vi "Serial Read to CRLF.vi"(8 "error in":errorcluster, 9 "timeout (ms)":i32, 10 "bytes to read":u32, 11 "Visa Resource":refnum<visa-resource-name>) -> (0 "error out":errorcluster, 1 "timed out?":bool, 3 "data":u8[](array[numeric]))   [LabVIEW 2021, in "Serial Shared Components.lvlib"]
doc: "Performs a read on the serial port."
uses:
  Serial Shared Components.lvlib
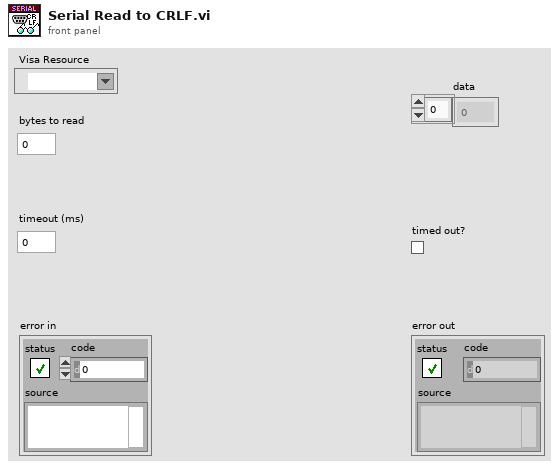
[diagram p1: front panel]
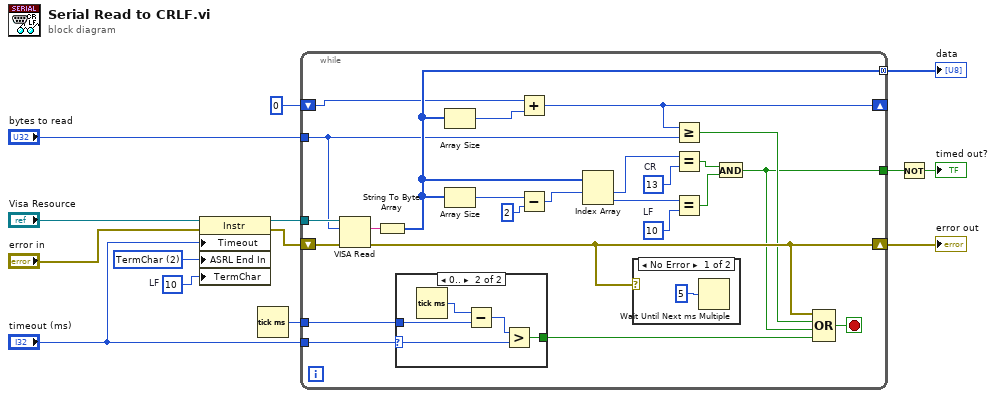
[diagram p0: block diagram]
diagram:
  w10 = u8 10  # LF
  w11 = u16 2 items=["None", "Last Bit", "TermChar"] ("Serial Settings:End Mode for Reads")
  n1 = property class="Instr"(reference="Visa Resource", error in="error in", "Timeout"="timeout (ms)", "ASRL End In"=w11, "TermChar"=w10) -> (reference out=w9:refnum<visa-resource-name>, error out=w8:errorcluster)
  n2 = Tick Count (ms)() -> (millisecond timer value=w13:u32)
  n3 = while {
    tunnel: w13 -> [w36]
    shift-right: [w34] -> w1
    shift-left: w8 -> [w38]
    tunnel: "bytes to read" -> [w22]
    tunnel: w9 -> [w35]
    tunnel: [w16] -> w3
    tunnel: "timeout (ms)" -> [w25]
    tunnel: [w24] -> w2 mode=concatenating
    shift-right: [w23] -> _
    shift-left: 0 -> [w18]
    stop <- w37 stop-if-true
    w28 = u8 10  # LF
    w15 = u8 13  # CR
    n4 = VISA Read(VISA resource name=w35, byte count=w22, error in (no error)=w38) -> (read buffer=w33:string, error out=w34:errorcluster)  [unwired: 2 out]
    n5 = String To Byte Array(string=w33) -> (unsigned byte array=w24:u8[])
    n6 = case shown="0.." w25 {
      selector: w25 -> [_ w39]
      tunnel: w36 -> [_ w42]
      tunnel: [_ w40] -> w21
      frame ..-1 {
        # "no t/o"
      }
      frame 0.. {
        n7 = Tick Count (ms)() -> (millisecond timer value=w43:u32)
        n8 = Subtract(x=w43, y=w42) -> (x-y=w41:u32)
        n9 = Greater?(x=w41, y=w39) -> (0:w40:bool)
      }
    }
    n10 = Array Size(array=w24) -> (size(s)=w19:i32)
    n11 = Array Size(array=w24) -> (size(s)=w32:i32)
    n12 = Add(x=w18, y=w19) -> (x+y=w23:i32)
    n13 = Subtract(x=w32, y=2) -> (x-y=w30:i32)
    n14 = Index Array(array=w24, index #1=w30) -> (element #1=w20:u8, element #2=w29:u8)  [unwired: 1 in]
    n15 = case shown="No Error" w34 {
      frame No Error {
        n16 = Wait Until Next ms Multiple(millisecond multiple=u32 5) -> ()  [unwired: 1 out]
      }
      frame Error {
      }
    }
    n17 = Greater Or Equal?(x=w23, y=w22) -> (x >= y?=w17:bool)
    n18 = Equal?(x=w20, y=w15) -> (x = y?=w26:bool)
    n19 = Equal?(x=w29, y=w28) -> (x = y?=w27:bool)
    n20 = And(x=w26, y=w27) -> (x .and. y?=w16:bool)
    n21 = Compound Arithmetic op=OR(w34, w17, w16, w21) -> (w37:bool)
  }
  "error out" <- w1
  "data" <- w2
  n22 = Not(x=w3) -> (.not. x?=→"timed out?":bool)
